vi "test passing.vi"(8 "error in (no error)":errorcluster, 11 "Dummy In":refnum<class "Dummy.lvclass">) -> (0 "error out":errorcluster, 3 "Dummy Out":refnum<class "Dummy.lvclass">)   [LabVIEW 2020, in "Dummy.lvclass"]
doc: "Passing test"
uses:
  Dummy.lvclass
  C:/git/astemes-lunit/source/API/LUnit Test Case/LUnit Test Case.lvclass
  API/LUnit Test Case/LUnit Test Case.lvclass/LUnit Test Case.ctl
  API/LUnit Test Case/Private/Append Fail Result.vi
  API/LUnit Test Case/Private/Append Pass Result.vi
  API/LUnit Test Case/LUnit Test Case.lvclass
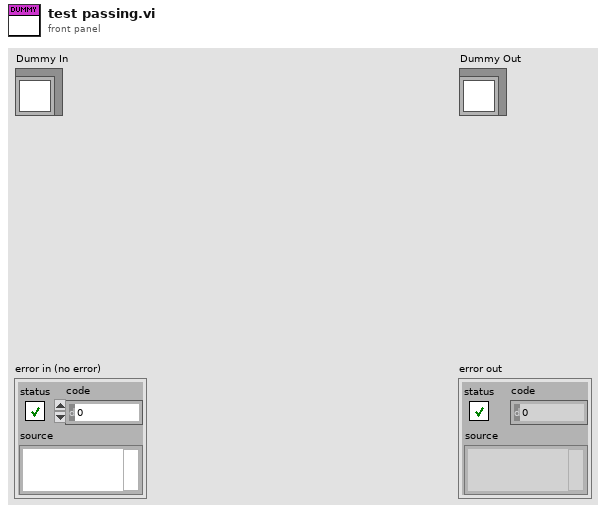
[diagram p1: front panel]
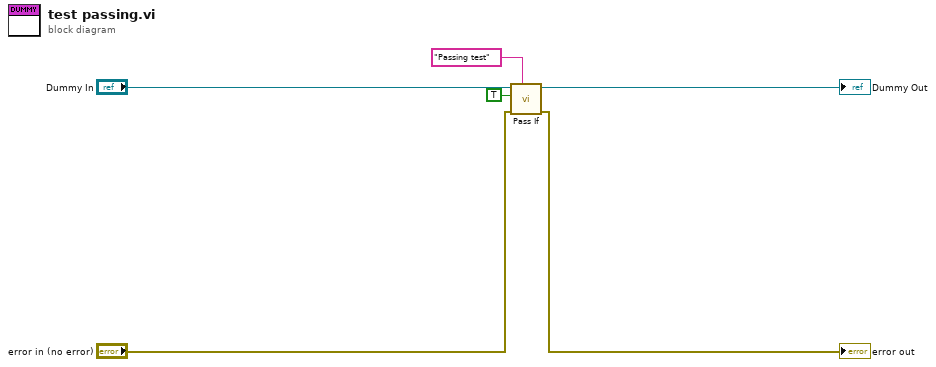
[diagram p0: block diagram]
diagram:
  n1 = call "Pass If.vi"("Description"="Passing test", "error in (no error)"="error in (no error)", "Pass?"=TRUE, "LUnit Test Case In"="Dummy In") -> ("error out"=→"error out":errorcluster, "LUnit Test Case Out"=→"Dummy Out":refnum<class "Dummy.lvclass">)  [unwired: 6 in]
